vi "Default or Users Font, Leading and Alignment.vi"(0 "PDF Report":T21(xcontrol), 5 "Font":T5={"Name"="", "Size"=-1.0, "Color"=0, "Style"={"Bold"=FALSE, "Italic"=FALSE, "Underline"=FALSE, "Strikeout"=FALSE}}, 9 "Paragraphe cluster":T1, 11 "error in (no error)":errorcluster) -> (4 "PDF Report duplicate":T21(xcontrol), 6 "Leading":T4=18.0, 8 "Font Ref":refnum<k24>, 10 "Close Font Ref":bool=TRUE, 14 "Aligment":string="JUSTIFY", 15 "error out":errorcluster)   [LabVIEW 2013]
doc: "Version 1.0\nDeveloped by Jean-Marc Simard\nCopyright © 2010, Exaprom Inc.\nAll rights reserved.\nLicense: BSD\n\nWith iTextSharp 4.1.6 (http://itextsharp.sourceforge.net)\nunder Mozilla Public License Version 1.1\n(http://www.mozilla.org/MPL/MPL-1.1.html)"
uses:
  Controls/PDF Report Xcontrol/PDF Report.xctl
  Controls/Font cluster.ctl
  Controls/Font size.ctl
  Controls/Font color.ctl
  C:/Users/MaxCorp/Documents/GitHub/TopView/DLL/itextsharp.dll
  DLL/itextsharp.dll
  Controls/Paragraphe cluster.ctl
  Controls/Texte alignement.ctl
  Controls/Line spacing.ctl
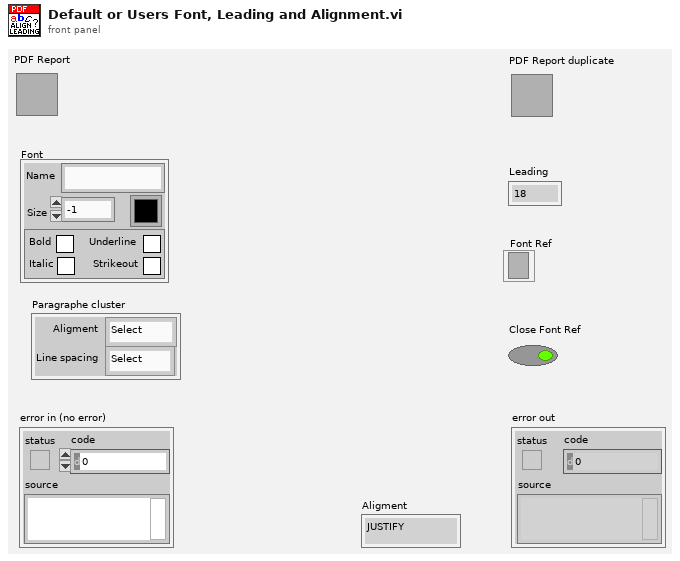
[diagram p1: front panel]
types:
  T1 = typedef "Paragraphe cluster.ctl" = cluster{" Aligment":T2, "Line spacing":T3}
  T2 = typedef "Texte alignement.ctl" = enum16{"Select", "CENTER", "JUSTIFY", "LEFT", "RIGHT"}
  T3 = typedef "Line spacing.ctl" = enum16{"Select", "1.0", "1.5", "2.0"}
  T4 = typedef "Font size.ctl" = sgl
  T5 = typedef "Font cluster.ctl" = cluster{"Name":string, "Size":T4, "Color":T6, "Style":cluster{"Bold":bool, "Italic":bool, "Underline":bool, "Strikeout":bool}}
  T6 = typedef "Font color.ctl" = u32
  T7 = typedef "Unit.ctl" = enum16{"inch", "mm"}
  T8 = typedef "Page dimensions.ctl" = cluster{"Start at page":i32, "Orientation":T9, "widht":sgl, "height":sgl, "Margin left":sgl, "Margin right":sgl, "Margin top":sgl, "Margin bottom":sgl}
  T9 = typedef "Page Orientation.ctl" = enum16{"Portrait", "Landscape"}
  T10 = typedef "Image or Table Caption.ctl" = cluster{"Caption":string, "Separator":string, "Position":enum16{"Above", "Below"}}
  T11 = typedef "Header Footer [ ].ctl" = T12[]
  T12 = typedef "Header Footer cluster.ctl" = cluster{"Start page":i32, "Type":T13, "Alignment":T14, "Vertical Alignement":T15, "Image (%)":sgl, "Page #":T16, "Text":string, "Path":string, "Font":T5, "Font refnum":refnum<k24>, "Line":cluster{"Line":T17, "Thickness (points)":sgl, "Colour":T6}}
  T13 = typedef "Header Footer Type.ctl" = enum16{"Select", "Text", "Text + hyperlink", "Page number", "Image", "Image + hyperlink"}
  T14 = typedef "Header footer horiz alignment.ctl" = enum16{"Left", "Center", "Right"}
  T15 = typedef "Cell Vertical alignment.ctl" = enum16{"TOP", "MIDDLE", "BOTTOM"}
  T16 = typedef "Page number.ctl" = cluster{"Text 1":string, "Text 2":string, "Text 3":string}
  T17 = typedef "Header Footer Line.ctl" = enum16{"No line", "Horizontal line"}
  T18 = typedef "Watermark cluster2.ctl" = cluster{"Show? (F)":bool, "Type":enum16{"Image", "Text"}, "Opacity (%)":sgl, "Rotate(°)":sgl, "Position":cluster{"Position":T19, "X":sgl, "Y":sgl}, "Image path":path, "Scaled(%)":sgl, "Image refnum":refnum<k24>, "Text":string, "Font":cluster{"Name":string, "Size":T4, "Color":T6}, "Font refnum":refnum<k24>, "Alignment":T14, "Automatic":bool}
  T19 = typedef "Watermark Position.ctl" = enum16{"Absolute", "Center (page)", "Center (text section)"}
  T20 = typedef "System Fonts.ctl" = cluster{"Font name [ ]":string[], "Font and file names [ ]":cluster{"Font name":string, "File name":string}[]}
  T21 = cluster{"Document":refnum<k24>, "Writer":refnum<k24>, "Default Font":refnum<k24>, "Default Font cluster":T5, "Path":path, "Unit (default = mm)":T7, "Paragraphe cluster":T1, "Pages dimensions [ ]":T8[], "Captions":cluster{"Image":T10, "Image counter":u16, "Table":T10, "Table counter":u16, "Font":T5}, "Header":T11, "Footer":T11, "Watermark ":T18, "Actual VI name":string, "System Fonts":T20}
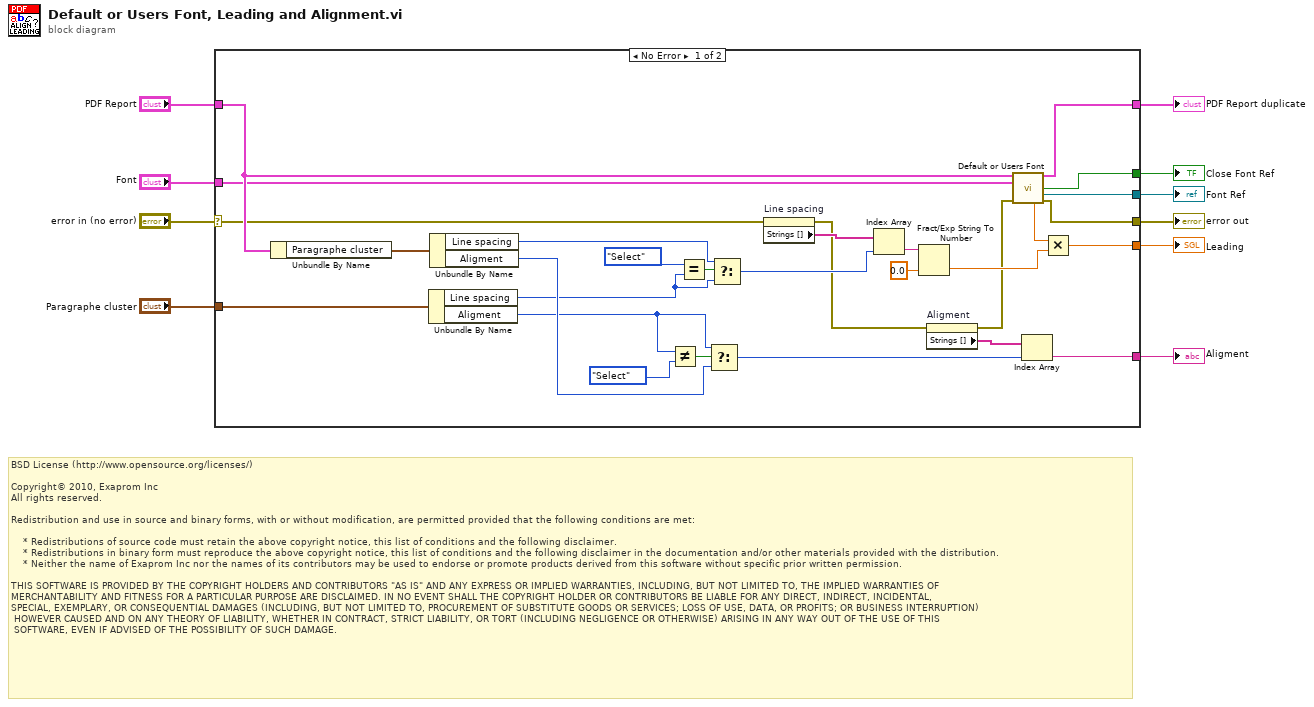
[diagram p0: block diagram]
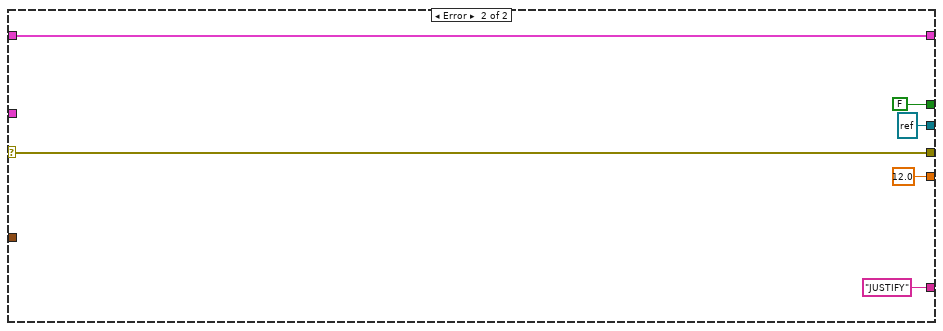
[diagram p2: hidden frame]
diagram:
  # "BSD License (http://www.opensource.org/licenses/)\n\nCopyright© 2010, Exaprom Inc\nAll rights reserved.\n\nRedistribution and use in source and binary forms, with or without modification, are permitted provided that the following conditions are met:\n\n    * Redistributions of source code must retain the above copyright notice, this list of conditions and the following disclaimer.\n    * Redistributions in binary form must reproduce the above copyright notice, this list of conditions and the following disclaimer in the documentation and/or other materials provided with the distribution.\n    * Neither the name of Exaprom Inc nor the names of its contributors may be used to endorse or promote products derived from this software without specific prior written permission.\n\nTHIS SOFTWARE IS PROVIDED BY THE COPYRIGHT HOLDERS AND CONTRIBUTORS \"AS IS\" AND ANY EXPRESS OR IMPLIED WARRANTIES, INCLUDING, BUT NOT LIMITED TO, THE IMPLIED WARRANTIES OF \nMERCHANTABILITY AND FITNESS FOR A PARTICULAR PURPOSE ARE DISCLAIMED. IN NO EVENT SHALL THE COPYRIGHT HOLDER OR CONTRIBUTORS BE LIABLE FOR ANY DIRECT, INDIRECT, INCIDENTAL,\nSPECIAL, EXEMPLARY, OR CONSEQUENTIAL DAMAGES (INCLUDING, BUT NOT LIMITED TO, PROCUREMENT OF SUBSTITUTE GOODS OR SERVICES; LOSS OF USE, DATA, OR PROFITS; OR BUSINESS INTERRUPTION)\n HOWEVER CAUSED AND ON ANY THEORY OF LIABILITY, WHETHER IN CONTRACT, STRICT LIABILITY, OR TORT (INCLUDING NEGLIGENCE OR OTHERWISE) ARISING IN ANY WAY OUT OF THE USE OF THIS\n SOFTWARE, EVEN IF ADVISED OF THE POSSIBILITY OF SUCH DAMAGE."
  n1 = case shown="No Error" "error in (no error)" {
    selector: "error in (no error)" -> [w11 w44]
    tunnel: [w39 "JUSTIFY"] -> w10
    tunnel: "Paragraphe cluster" -> [w38 _]
    tunnel: [w20 T4 12.0 ("Font Size")] -> w8
    tunnel: "PDF Report" -> [w19 w45]
    tunnel: [w18 w45] -> w6
    tunnel: "Font" -> [w17 _]
    tunnel: [w16 FALSE ("Close Font Ref")] -> w4
    tunnel: [w15 refnum<k24> refnum ("Font Ref")] -> w3
    tunnel: [w12 w44] -> w2
    frame No Error {
      n2 = Unbundle By Name(w19) -> ("Paragraphe cluster"=w22:T1)
      n3 = Unbundle By Name(w38) -> ("Line spacing"=w28:T3, "Aligment"=w27:T2)
      n4 = Unbundle By Name(w22) -> ("Line spacing"=w30:T3, "Aligment"=w29:T2)
      n5 = Not Equal?(x=w27, y=Texte_alignement."Select" ("Aligment 2")) -> (x != y?=w32:bool)
      n6 = Equal?(x=Line_spacing."Select", y=w28) -> (x = y?=w34:bool)
      n7 = Select(t=w27, s=w32, f=w29) -> (s? t:f=w31:T2)
      n8 = Select(t=w30, s=w34, f=w28) -> (s? t:f=w33:T3)
      n9 = property on="Line spacing" class="Enum (strict)"(error in=w11) -> (error out=w24:errorcluster, "Strings []"=w25:string[])  [unwired: 1 in, 1 out]
      n10 = Index Array(array=w25, index=w33) -> (element=w36:string)
      n11 = Fract/Exp String To Number(string=w36, default (0 dbl)=sgl 0.0 ("default (0 DBL)")) -> (number=w21:sgl)  [unwired: 3 out]
      n12 = property on="Aligment" class="Enum (strict)"(error in=w24) -> (error out=w13:errorcluster, "Strings []"=w23:string[])  [unwired: 1 in, 1 out]
      n13 = call "Default or Users Font.vi"("PDF Report"=w19, "Font"=w17, "error in (no error)"=w13) -> ("PDF Report duplicate"=w18:T21, "Close Font Ref"=w16:bool, "Font Ref"=w15:refnum<k24>, "Font Size"=w14:T4, "error out"=w12:errorcluster)  [unwired: 8 out]
      n14 = Index Array(array=w23, index=w31) -> (element=w39:string)
      n15 = Multiply(x=w14, y=w21) -> (x*y=w20:T4)
    }
    frame Error {
    }
  }
  "PDF Report duplicate" <- w6
  "error out" <- w2
  "Font Ref" <- w3
  "Leading" <- w8
  "Aligment" <- w10
  "Close Font Ref" <- w4
